vi "Simple Example.vi"() -> ()   [LabVIEW 2020]
uses:
  C:/GEECS/Developers Version/builds/Device builds/ThorlabsKCube_InertialMotor/Thorlabs.MotionControl.KCube.InertialMotorCLI.dll
  Thorlabs.MotionControl.KCube.InertialMotorCLI.dll
  C:/GEECS/Developers Version/builds/Device builds/ThorlabsKCube_InertialMotor/Thorlabs.MotionControl.Controls.dll
  Thorlabs.MotionControl.Controls.dll
panel:
  out "Array":i32[](array[numeric])
  in  "Get all Positions":bool
  in  "Boolean":bool
  in  "Set Enable":bool
  out "IsAnyChannelMoving":bool
  in  "Set Abort":bool
  in  "Move to":dbl
  in  "Set Position":bool
  in  "Channel":i8
  in  "Get Position":bool
  in  "stop":bool
  out "GetPosition":i32
  out "error out":errorcluster
  in  "SerialNumber":string
  in  "KCubeInertialMotorControl":refnum<k24>(container)
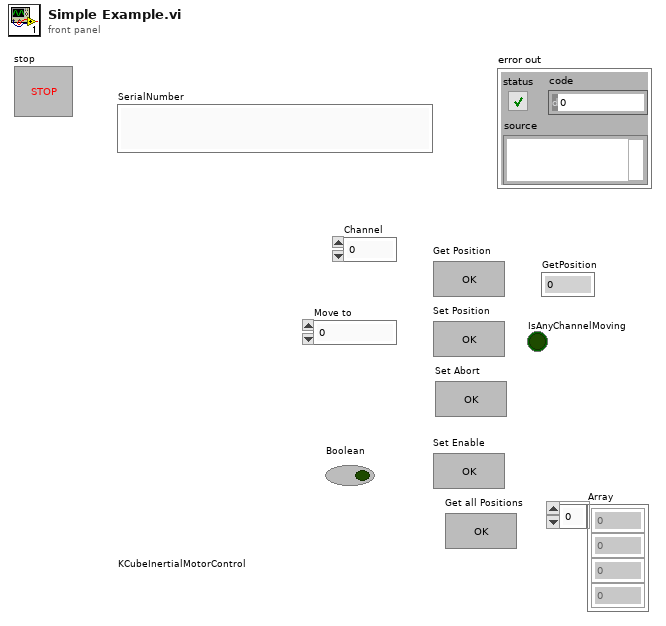
[diagram p1: front panel]
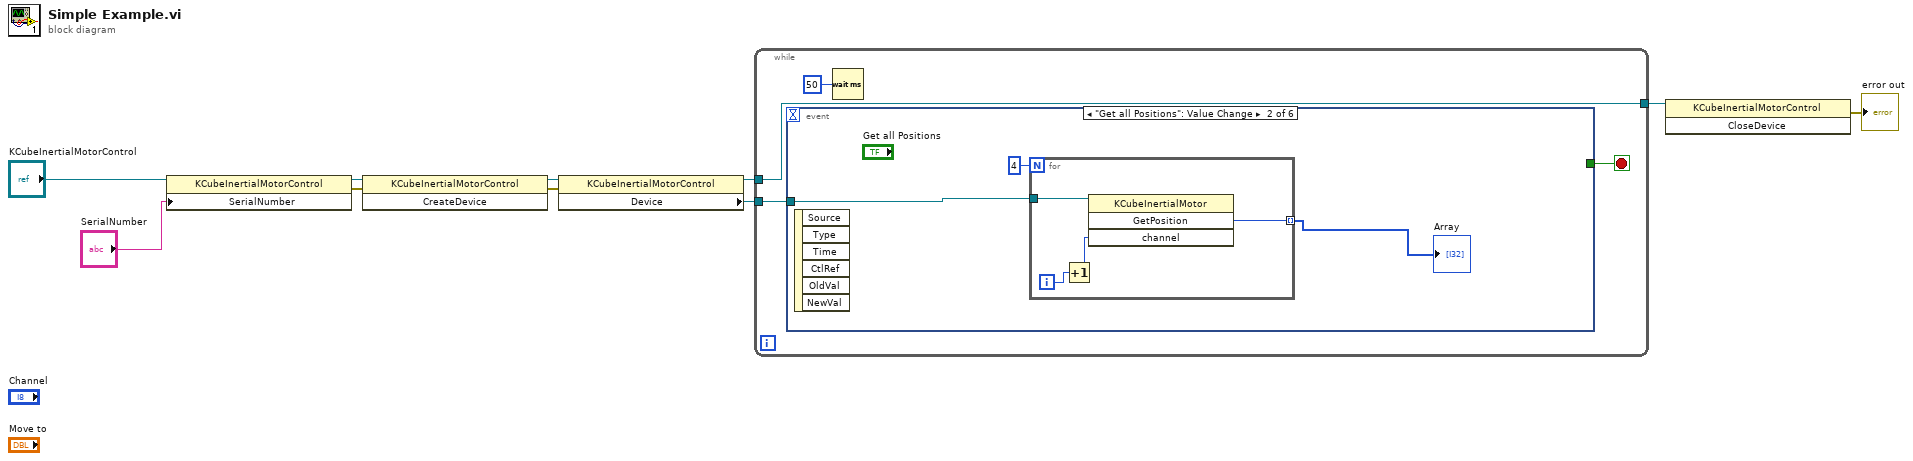
[diagram p0: block diagram]
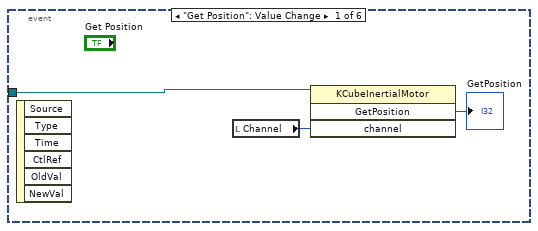
[diagram p2: hidden frame]
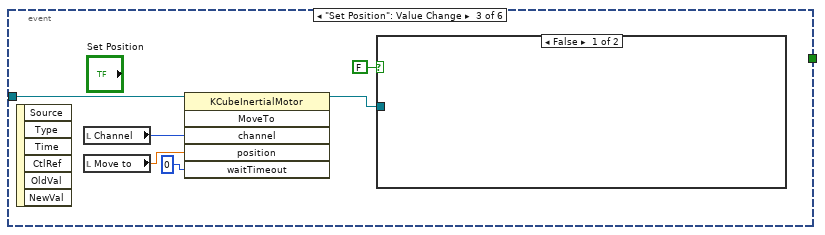
[diagram p3: hidden frame]
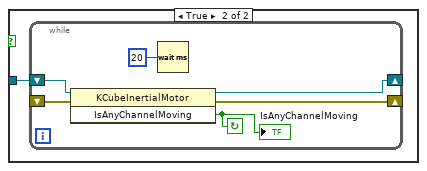
[diagram p4: hidden frame]
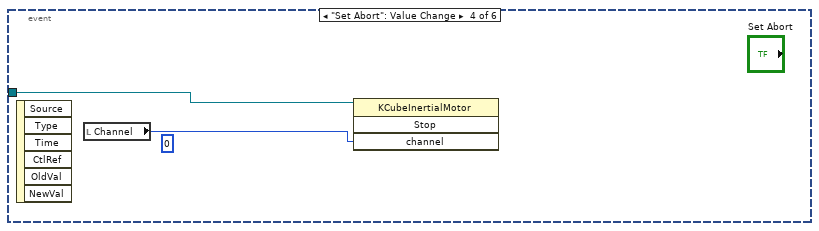
[diagram p5: hidden frame]
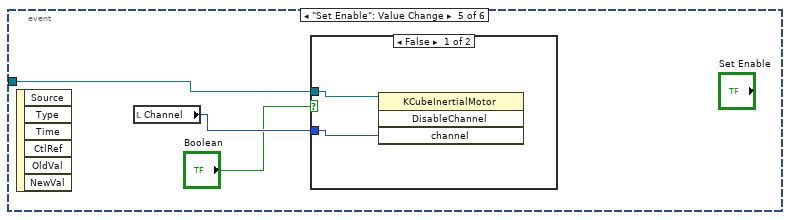
[diagram p6: hidden frame]
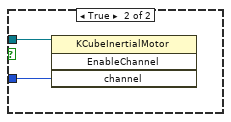
[diagram p7: hidden frame]
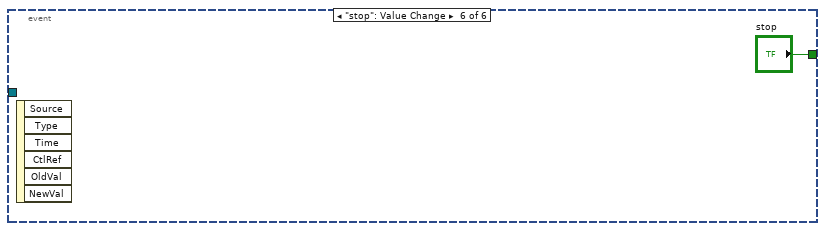
[diagram p8: hidden frame]
diagram:
  n1 = property class="KCubeInertialMotorControl"(reference="KCubeInertialMotorControl", "SerialNumber"="SerialNumber") -> (reference out=w8:refnum<k24>, error out=w6:errorcluster)  [unwired: 1 in]
  n2 = invoke class="KCubeInertialMotorControl" method="CreateDevice"(reference=w8, error in=w6) -> (reference out=w7:refnum<k24>, error out=w5:errorcluster)  [unwired: 1 in, 1 out]
  n3 = property class="KCubeInertialMotorControl"(reference=w7, error in=w5) -> (reference out=w3:refnum<k24>, "Device"=w1:refnum<k24>)  [unwired: 1 out]
  n4 = while {
    tunnel: w3 -> [w14]
    tunnel: [w14] -> w2
    tunnel: w1 -> [w13]
    stop <- w11 stop-if-true
    n5 = event shown="[1] \"Get all Positions\": Value Change" {
      selector: _ -> [_ _ _ _ _ _]
      dyn-events: _ -> [_ _ _ _ _ _]
      timeout: _ -> [_ _ _ _ _ _]
      tunnel: w13 -> [w17 w20 w30 w39 w42 _]
      tunnel: [_ _ _ _ _ "stop"] -> w11
      event "Get Position": Value Change {
        n6 = event-data() -> ()  [unwired: 1 in, 6 out]
        n7 = local read "Channel"() -> (w15:i8)
        n8 = invoke class="KCubeInertialMotor" method="GetPosition"(reference=w17, "channel"=w15) -> ("GetPosition"=→"GetPosition":i32)  [unwired: 2 in, 3 out]
      }
      event "Get all Positions": Value Change {
        n9 = event-data() -> ()  [unwired: 1 in, 6 out]
        n10 = for {
          N: 4 -> [_]
          tunnel: w20 -> [w24]
          tunnel: [w23] -> w19 mode=indexing
          i -> [w22]
          n11 = Increment(x=w22) -> (x+1=w21:i32)
          n12 = invoke class="KCubeInertialMotor" method="GetPosition"(reference=w24, "channel"=w21) -> ("GetPosition"=w23:i32)  [unwired: 2 in, 3 out]
        }
        "Array" <- w19
      }
      event "Set Position": Value Change {
        n13 = event-data() -> ()  [unwired: 1 in, 6 out]
        n14 = local read "Channel"() -> (w29:i8)
        n15 = local read "Move to"() -> (w27:dbl)
        n16 = invoke class="KCubeInertialMotor" method="MoveTo"(reference=w30, "channel"=w29, "position"=w27, "waitTimeout"=0) -> (reference out=w26:refnum<k24>)  [unwired: 2 in, 5 out]
        n17 = case shown="False" FALSE {
          tunnel: w26 -> [_ w31]
          frame False {
          }
          frame True {
            n18 = while {
              shift-right: [w36] -> _
              shift-left: _ -> [w37]
              shift-right: [w34] -> _
              shift-left: w31 -> [w35]
              stop <- w32 continue-if-true
              n19 = invoke class="KCubeInertialMotor" method="IsAnyChannelMoving"(reference=w35, error in=w37) -> (reference out=w34:refnum<k24>, error out=w36:errorcluster, "IsAnyChannelMoving"=w32:bool)  [unwired: 1 in]
              "IsAnyChannelMoving" <- w32
              n20 = Wait (ms)(milliseconds to wait=u32 20) -> ()  [unwired: 1 out]
            }
          }
        }
      }
      event "Set Abort": Value Change {
        (unwired) 0 ("waitTimeout")
        n21 = event-data() -> ()  [unwired: 1 in, 6 out]
        n22 = local read "Channel"() -> (w38:i8)
        n23 = invoke class="KCubeInertialMotor" method="Stop"(reference=w39, "channel"=w38) -> ()  [unwired: 2 in, 4 out]
      }
      event "Set Enable": Value Change {
        n24 = event-data() -> ()  [unwired: 1 in, 6 out]
        n25 = local read "Channel"() -> (w41:i8)
        n26 = case shown="False" "Boolean" {
          tunnel: w42 -> [w44 w46]
          tunnel: w41 -> [w43 w45]
          frame False {
            n27 = invoke class="KCubeInertialMotor" method="DisableChannel"(reference=w44, "channel"=w43) -> ()  [unwired: 2 in, 4 out]
          }
          frame True {
            n28 = invoke class="KCubeInertialMotor" method="EnableChannel"(reference=w46, "channel"=w45) -> ()  [unwired: 2 in, 4 out]
          }
        }
      }
      event "stop": Value Change {
        n29 = event-data() -> ()  [unwired: 1 in, 6 out]
      }
    }
    n30 = Wait (ms)(milliseconds to wait=u32 50) -> ()  [unwired: 1 out]
  }
  n31 = invoke class="KCubeInertialMotorControl" method="CloseDevice"(reference=w2) -> (error out=→"error out":errorcluster)  [unwired: 2 in, 2 out]
